vi "GPS Test Read.vi"() -> ()   [LabVIEW 2009]
uses:
  <vilib>/Instr/_visa.llb/VISA Configure Serial Port (Instr).vi
panel:
  out "Output Started":bool
  out "Error Out":errorcluster
  out "Output Halted":bool
  in  "stop":bool
  in  "Mode":enum16{"VISA", "Simulate SubVI"}(ring)
  out "Latitude":dbl
  out "Time":dbl
  out "Longitude":dbl
  out "Buffer Out":string
  in  "VISA resource name":refnum<visa-resource-name>="COM1"
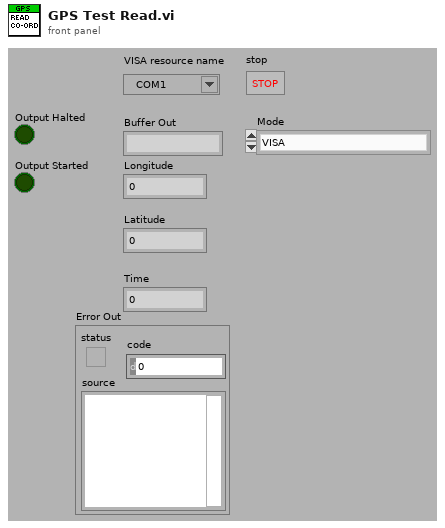
[diagram p1: front panel]
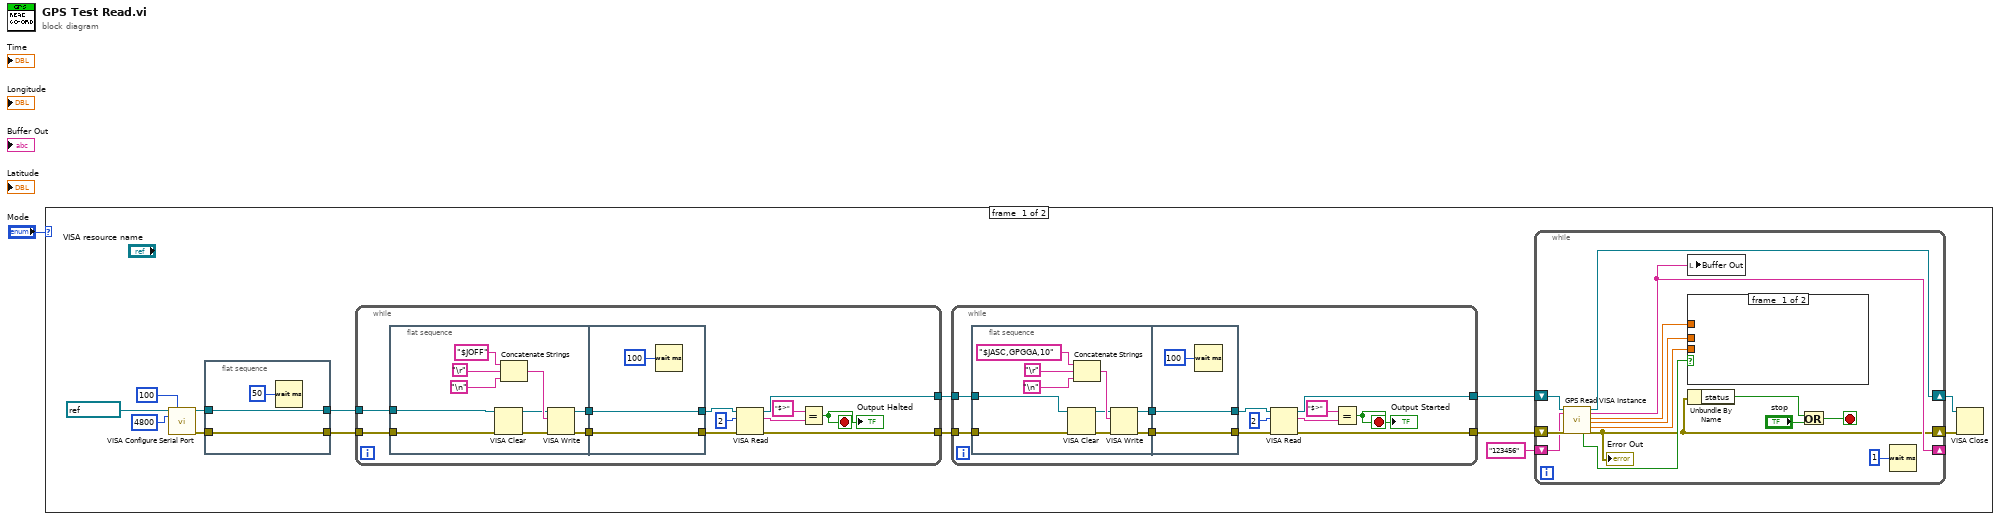
[diagram p0: block diagram]
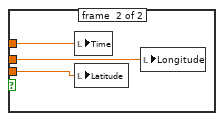
[diagram p2: hidden frame]
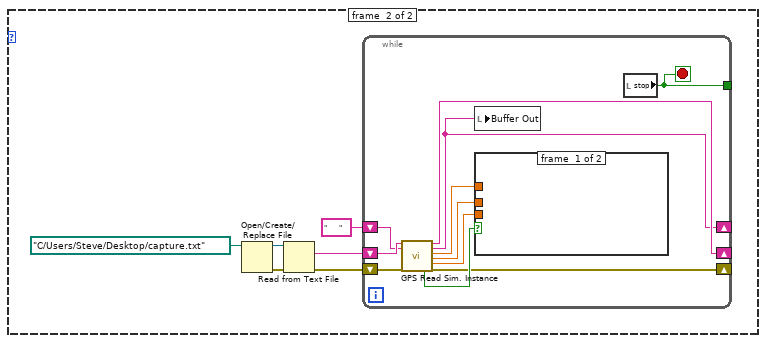
[diagram p3: hidden frame]
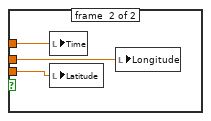
[diagram p4: hidden frame]
diagram:
  n1 = case shown="\"VISA\", Default" "Mode" {
    frame #0 {
      n2 = call-poly "VISA Configure Serial Port"("VISA resource name"=refnum<visa-resource-name> "COM1", "timeout (10sec)"=u32 100, "baud rate (9600)"=u32 4800) -> ("VISA resource name out"=w8:refnum<visa-resource-name>, "error out"=w10:errorcluster)  [unwired: 11 in]
      n3 = flat-sequence {
        tunnel: [w66] -> w7
        tunnel: w10 -> [w66]
        tunnel: w8 -> [w67]
        tunnel: [w67] -> w6
        frame #0 {
          n4 = Wait (ms)(milliseconds to wait=u32 50) -> ()  [unwired: 1 out]
        }
      }
      n5 = while {
        tunnel: w7 -> [w52]
        tunnel: w6 -> [w51]
        tunnel: [w46] -> w4
        tunnel: [w45] -> w5
        stop <- w47 stop-if-true
        n6 = flat-sequence {
          tunnel: w52 -> [w62]
          tunnel: w51 -> [w61]
          tunnel: [w56] -> w43
          tunnel: [w53] -> w41
          tunnel: [w64] -> w44
          tunnel: w43 -> [w64]
          tunnel: [w63] -> w42
          tunnel: w41 -> [w63]
          frame #0 {
            n7 = VISA Clear(VISA resource name=w61, error in (no error)=w62) -> (VISA resource name out=w54:refnum<visa-resource-name>, error out=w55:errorcluster)
            n8 = Concatenate Strings("$JOFF" ("Ascii to write 2"), "\r", "\n") -> (w59:string)
            n9 = VISA Write(VISA resource name=w54, write buffer=w59, error in (no error)=w55) -> (VISA resource name out=w53:refnum<visa-resource-name>, error out=w56:errorcluster)  [unwired: 1 out]
          }
          frame #1 {
            n10 = Wait (ms)(milliseconds to wait=u32 100) -> ()  [unwired: 1 out]
          }
        }
        n11 = VISA Read(VISA resource name=w42, byte count=u32 2, error in (no error)=w44) -> (VISA resource name out=w45:refnum<visa-resource-name>, read buffer=w49:string, error out=w46:errorcluster)  [unwired: 1 out]
        n12 = Equal?(x="$>" ("read buffer"), y=w49) -> (x = y?=w47:bool)
        "Output Halted" <- w47
      }
      n13 = while {
        tunnel: w4 -> [w27]
        tunnel: w5 -> [w26]
        tunnel: [w21] -> w3
        tunnel: [w20] -> w2
        stop <- w22 stop-if-true
        n14 = flat-sequence {
          tunnel: w27 -> [w37]
          tunnel: w26 -> [w36]
          tunnel: [w31] -> w18
          tunnel: [w28] -> w16
          tunnel: [w39] -> w19
          tunnel: w18 -> [w39]
          tunnel: [w38] -> w17
          tunnel: w16 -> [w38]
          frame #0 {
            n15 = VISA Clear(VISA resource name=w36, error in (no error)=w37) -> (VISA resource name out=w29:refnum<visa-resource-name>, error out=w30:errorcluster)
            n16 = Concatenate Strings("$JASC,GPGGA,10" ("Ascii to write 2"), "\r", "\n") -> (w34:string)
            n17 = VISA Write(VISA resource name=w29, write buffer=w34, error in (no error)=w30) -> (VISA resource name out=w28:refnum<visa-resource-name>, error out=w31:errorcluster)  [unwired: 1 out]
          }
          frame #1 {
            n18 = Wait (ms)(milliseconds to wait=u32 100) -> ()  [unwired: 1 out]
          }
        }
        n19 = VISA Read(VISA resource name=w17, byte count=u32 2, error in (no error)=w19) -> (VISA resource name out=w20:refnum<visa-resource-name>, read buffer=w24:string, error out=w21:errorcluster)  [unwired: 1 out]
        n20 = Equal?(x="$>" ("read buffer"), y=w24) -> (x = y?=w22:bool)
        "Output Started" <- w22
      }
      n21 = while {
        shift-right: [w75] -> _
        shift-left: "123456" ("String") -> [w76]
        shift-right: [w70] -> w13
        shift-left: w3 -> [w81]
        shift-right: [w82] -> w14
        shift-left: w2 -> [w80]
        stop <- w71 stop-if-true
        n22 = call "GPS Read VISA Instance.vi"("VISA In"=w80, "Buffer In"=w76, "Error In"=w81) -> ("Output Valid?"=w74:bool, "VISA Out"=w82:refnum<visa-resource-name>, "Buffer Out"=w75:string, "Time"=w77:dbl, "Longitude"=w79:dbl, "Latitude"=w78:dbl, "Error Out"=w70:errorcluster)  [unwired: 10 in]
        "Error Out" <- w70
        n23 = local write "Buffer Out"(w75) -> ()
        n24 = case shown="True" w74 {
          tunnel: w79 -> [_ w84]
          tunnel: w78 -> [_ w83]
          tunnel: w77 -> [_ w85]
          frame #0 {
          }
          frame #1 {
            n25 = local write "Time"(w85) -> ()
            n26 = local write "Latitude"(w83) -> ()
            n27 = local write "Longitude"(w84) -> ()
          }
        }
        n28 = Unbundle By Name(w70) -> ("status"=w69:bool)
        n29 = Or(x=w69, y="stop") -> (x .or. y?=w71:bool)
        n30 = Wait (ms)(milliseconds to wait=u32 1) -> ()  [unwired: 1 out]
      }
      n31 = VISA Close(VISA resource name=w14, error in (no error)=w13) -> ()  [unwired: 1 out]
    }
    frame #1 {
      n32 = Open/Create/Replace File(file path (use dialog)=path "C:/Users/Steve/Desktop/capture.txt" ("file (use dialog)")) -> (refnum out=w86:refnum<file>, error out=w89:errorcluster)  [unwired: 5 in, 1 out]
      n33 = Read from Text File(file (use dialog)=w86, error in=w89) -> (text=w88:string, error out=w87:errorcluster)  [unwired: 2 in, 2 out]
      n34 = while {
        shift-right: [w97] -> _
        shift-left: "      " ("String") -> [w100]
        tunnel: [w102] -> _
        shift-right: [w92] -> _
        shift-left: w87 -> [w99]
        shift-right: [w98] -> _
        shift-left: w88 -> [w101]
        stop <- w102 stop-if-true
        n35 = call "GPS Read Sim. Instance.vi"("String In"=w101, "Buffer In"=w100, "error in (no error)"=w99) -> ("Output Valid"=w93:bool, "String Out"=w98:string, "Buffer Out"=w97:string, "Time"=w96:dbl, "Longitude"=w95:dbl, "Latitude"=w94:dbl, "error out"=w92:errorcluster)  [unwired: 10 in]
        n36 = local write "Buffer Out"(w97) -> ()
        n37 = case shown="True" w93 {
          tunnel: w95 -> [_ w104]
          tunnel: w94 -> [_ w103]
          tunnel: w96 -> [_ w105]
          frame #0 {
          }
          frame #1 {
            n38 = local write "Time"(w105) -> ()
            n39 = local write "Latitude"(w103) -> ()
            n40 = local write "Longitude"(w104) -> ()
          }
        }
        n41 = local read "stop"() -> (w102:bool)
      }
    }
  }
